vi "Model - DeInit.vi"(8 "error in (no error)":errorcluster, 11 "View Model":T1) -> (0 "error out":errorcluster)   [LabVIEW 2017]
doc: "De-Initialize all components of View Model"
uses:
  Controls/View Model.ctl
  Controls/Shared Model.ctl
  Error Handler/Controls/Error Model.ctl
  Error Handler/Controls/Error Event.ctl
  Error Handler/Controls/Error Type.ctl
  Controller/Controls/Controller Model.ctl
  Controller/Controls/Controller Event.ctl
  Controller/Controls/Controller Command.ctl
  Controller/Controls/Controller Overhead.ctl
  Real-Time/RT Status.ctl
  Real-Time/RT Loop Status.ctl
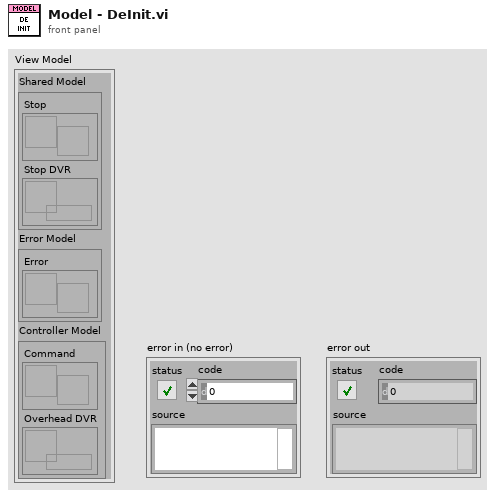
[diagram p1: front panel]
types:
  T1 = typedef "View Model.ctl" = cluster{"Shared Model":T2, "Error Model":T3, "Controller Model":T4}
  T2 = typedef "Shared Model.ctl" = cluster{"Stop":refnum<user-event>, "Stop DVR":refnum<data-value>}
  T3 = typedef "Error Model.ctl" = cluster{"Error":refnum<user-event>}
  T4 = typedef "Controller Model.ctl" = cluster{"Command":refnum<user-event>, "Overhead DVR":refnum<data-value>}
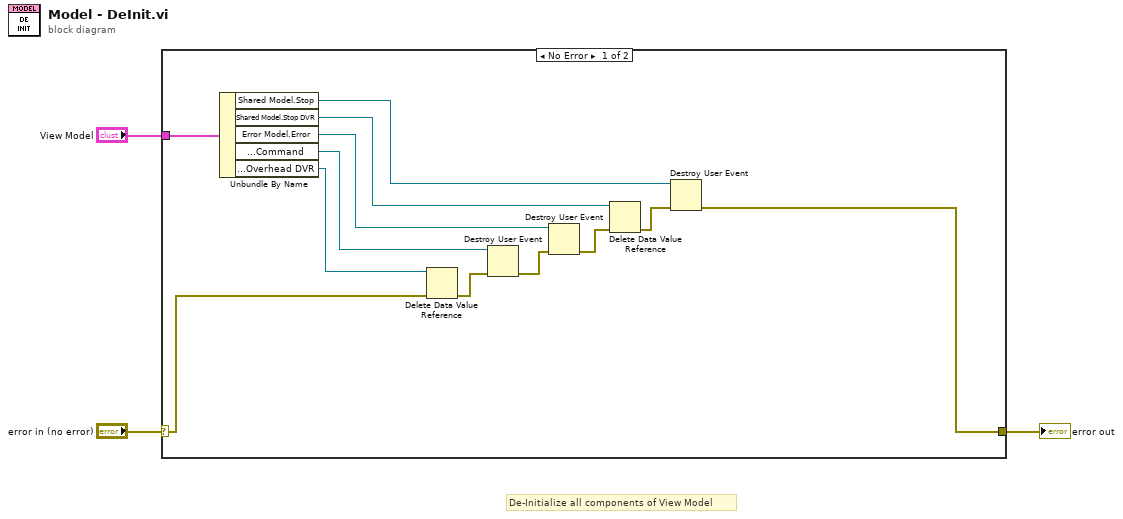
[diagram p0: block diagram]
diagram:
  # "De-Initialize all components of View Model"
  n1 = case shown="No Error" "error in (no error)" {
    selector: "error in (no error)" -> [w5 w16]
    tunnel: [w4 w16] -> w2
    tunnel: "View Model" -> [w15 _]
    frame No Error {
      n2 = Unbundle By Name(w15) -> ("Shared Model.Stop"=w6:refnum<user-event>, "Shared Model.Stop DVR"=w8:refnum<data-value>, "Error Model.Error"=w11:refnum<user-event>, "Controller Model.Command"=w12:refnum<user-event>, "Controller Model.Overhead DVR"=w14:refnum<data-value>)
      n3 = Delete Data Value Reference(data value reference=w14, error in=w5) -> (error out=w13:errorcluster)  [unwired: 1 out]
      n4 = Destroy User Event(user event=w12, error in=w13) -> (error out=w10:errorcluster)
      n5 = Destroy User Event(user event=w11, error in=w10) -> (error out=w9:errorcluster)
      n6 = Delete Data Value Reference(data value reference=w8, error in=w9) -> (error out=w7:errorcluster)  [unwired: 1 out]
      n7 = Destroy User Event(user event=w6, error in=w7) -> (error out=w4:errorcluster)
    }
    frame Error {
    }
  }
  "error out" <- w2
